vi "Draw Paq Disp FP.vi"(10 "This VI Paq Disp":refnum<vi>, 11 "Sub Panel Paq Disp":refnum<vi>) -> ()   [LabVIEW 2020, in "Paquetes Disponibles.lvlib"]
uses:
  Paquetes Disponibles.lvlib
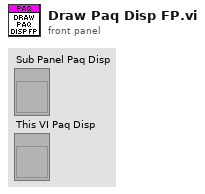
[diagram p1: front panel]
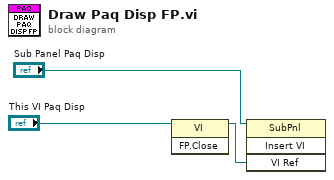
[diagram p0: block diagram]
diagram:
  n1 = invoke class="VI" method="FP.Close"(reference="This VI Paq Disp") -> (reference out=w3:refnum<vi>)  [unwired: 2 in, 2 out]
  n2 = invoke class="SubPnl" method="Insert VI"(reference="Sub Panel Paq Disp", "VI Ref"=w3) -> ()  [unwired: 2 in, 4 out]
